vi "ex_4.vi"() -> ()   [LabVIEW 2020]
uses:
  #typedef_FGV_TimerAction_ex_4.ctl
panel:
  in  "stop":bool
  in  "Timer action (run)":T1=enum."Run"
  out "Time Elapsed":dbl
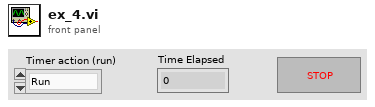
[diagram p1: front panel]
types:
  T1 = typedef "#typedef_FGV_TimerAction_ex_4.ctl" = enum16{"Reset", "Run", "Pause"}
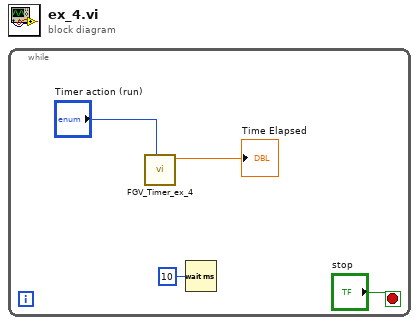
[diagram p0: block diagram]
diagram:
  n1 = while {
    stop <- "stop" stop-if-true
    n2 = call "FGV_Timer_ex_4.vi"("Timer action (run)"="Timer action (run)") -> ("Time Elapsed"=→"Time Elapsed":dbl)  [unwired: 9 in, 1 out]
    n3 = Wait (ms)(milliseconds to wait=u32 10) -> ()  [unwired: 1 out]
  }
